vi "LabViewDllTest.vi"() -> ()   [LabVIEW 2017]
panel:
  out "size(s)":i32
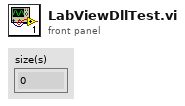
[diagram p1: front panel]
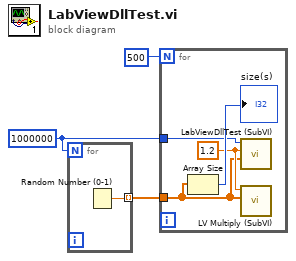
[diagram p0: block diagram]
diagram:
  w1 = 1000000
  n1 = for {
    N: w1 -> [_]
    tunnel: [w4] -> w2 mode=indexing
    n2 = Random Number (0-1)() -> (number: 0 to 1=w4:dbl)
  }
  n3 = for {
    N: 500 -> [_]
    tunnel: w2 -> [w6]
    tunnel: w1 -> [w5]
    w7 = 1.2 ("c")
    n4 = Array Size(array=w6) -> (size(s)=→"size(s)":i32)
    n5 = call "LabViewDllTest (SubVI).vi"("Array"=w6, "c"=w7, "Numeric"=w5) -> ()  [unwired: 7 in, 2 out]
    n6 = call "LV Multiply (SubVI).vi"("Array in"=w6, "c"=w7) -> ()  [unwired: 9 in, 1 out]
  }
